vi "DSF.Engine.Transceiver Thread.Tx.vi"(8 "error in (no error)":errorcluster, 10 "Transfer Group in":refnum<class "DSF.Engine.Transfer Group.lvclass">, 11 "Transceiver Thread in":refnum<class "DSF.Engine.Transceiver Thread.lvclass">) -> (0 "error out":errorcluster, 2 "Transfer Group out":refnum<class "DSF.Engine.Transfer Group.lvclass">, 3 "Transceiver Thread out":refnum<class "DSF.Engine.Transceiver Thread.lvclass">)   [LabVIEW 2017, in "Data Sharing Framework Engine.lvlib" / "DSF.Engine.Transceiver Thread.lvclass"]
uses:
  DSF.Engine.Transceiver Thread.lvclass
  Transfer/DSF.Engine.Transfer Group.lvclass
  DSF.Engine.Transceiver Thread.lvclass/DSF.Engine.Transceiver Thread.ctl
  DSF.Engine.Transceiver.lvclass
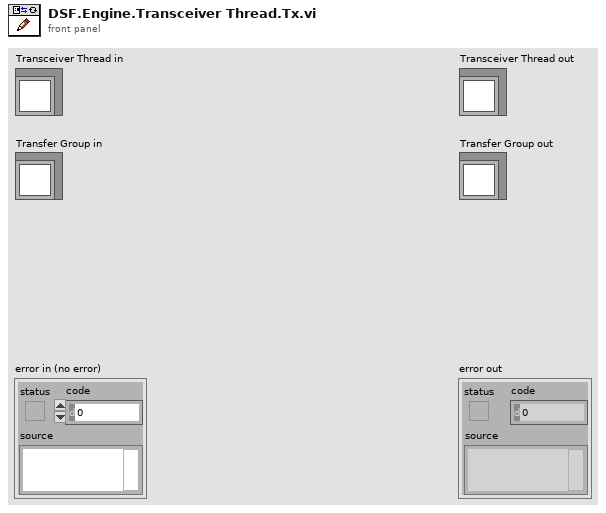
[diagram p1: front panel]
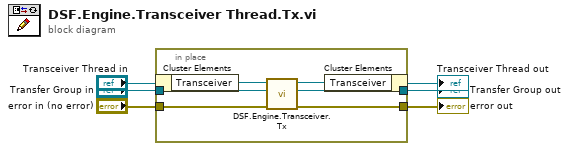
[diagram p0: block diagram]
diagram:
  n1 = in-place {
    in-place-border: "error in (no error)" -> [w12]
    in-place-border: "Transfer Group in" -> [w11]
    in-place-border: [w10] -> w3
    in-place-border: [w9] -> w2
    n2 = in-place-cluster #1("Transceiver Thread in") -> ("Transceiver"=w8:refnum<class "DSF.Engine.Transceiver.lvclass">)
    n3 = call-dynamic "DSF.Engine.Transceiver.Tx.vi"("error in (no error)"=w12, "Transfer Group in"=w11, "Transceiver in"=w8) -> ("error out"=w10:errorcluster, "Transfer Group out"=w9:refnum<class "DSF.Engine.Transfer Group.lvclass">, "Transceiver out"=w7:refnum<class "DSF.Engine.Transceiver.lvclass">)  [unwired: 6 in]
    n4 = in-place-cluster #1("Transceiver"=w7) -> (→"Transceiver Thread out":refnum<class "DSF.Engine.Transceiver Thread.lvclass">)
  }
  "error out" <- w3
  "Transfer Group out" <- w2
